vi "Acquire Start Msg.vi"(8 "error in (no error)":errorcluster, 11 "Message Queues in":T1) -> (0 "error out":errorcluster, 3 "Message Queues out":T1)   [LabVIEW 2018, in "Message Queue.lvlib"]
uses:
  Message Queue.lvlib
  All Message Queues.ctl
  Message Cluster.ctl
  Controls/Data Queue.ctl
  Controls/Acquired Data.ctl
  Controls/Data Notifier.ctl
  Enqueue Message (Single).vi
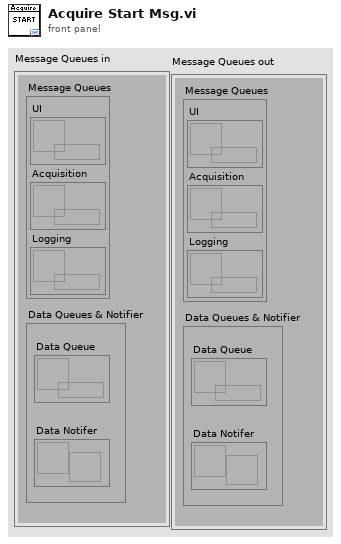
[diagram p1: front panel]
types:
  T1 = typedef "Message Queue.lvlib/All Message Queues.ctl" = cluster{"Message Queues":cluster{"UI":refnum<queue>, "Acquisition":refnum<queue>, "Logging":refnum<queue>}, "Data Queues & Notifier":cluster{"Data Queue":T2, "Data Notifer":T3}}
  T2 = typedef "Data Queue.ctl" = refnum<queue>
  T3 = typedef "Data Notifier.ctl" = refnum<notifier>
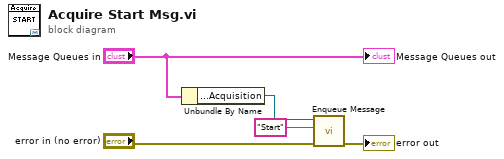
[diagram p0: block diagram]
diagram:
  n1 = Unbundle By Name("Message Queues in") -> ("Message Queues.Acquisition"=w1:refnum<queue>)
  n2 = call-poly "Enqueue Message.vi"("error in (no error)"="error in (no error)", "Message"="Start", "Message Queue"=w1) -> ("error out"=→"error out":errorcluster)  [unwired: 7 in, 1 out]
  "Message Queues out" <- "Message Queues in"
